vi "Untitled 3.vi"   [LabVIEW 2020]
uses:
  Global 1.vi
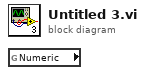
[diagram p0: block diagram]
diagram:
  n1 = global read "Global 1.vi" "Numeric"() -> ()  [unwired: 1 out]
